vi "IMP Driver.vi"(5 "IMP Driver (\"\")":string, 6 "Drv Refnum":T1, 7 "IMP Command":T2, 8 "error in (no error)":errorcluster, 11 "Variant Input":variant) -> (0 "error out":errorcluster, 3 "Variant Output":variant, 4 "dup Drv Refnum":T1)   [LabVIEW 2011]
uses:
  IMP Command.ctl
  IMP Driver Ref.ctl
panel:
  in  "DEBUG?":bool
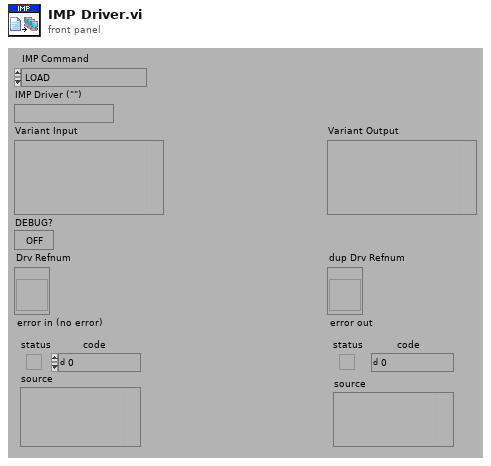
[diagram p1: front panel]
types:
  T1 = typedef "IMP Driver Ref.ctl" = refnum<vi>
  T2 = typedef "IMP Command.ctl" = enum16{"LOAD", "INITIALIZE", "IMPORT", "UNLOAD"}
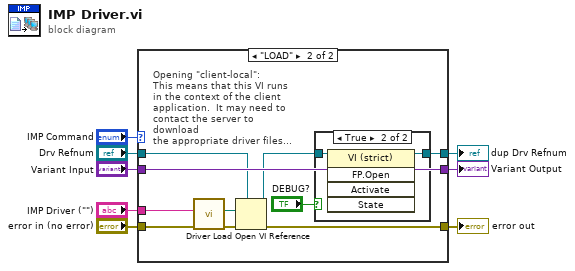
[diagram p0: block diagram]
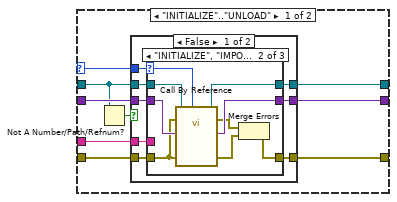
[diagram p2: hidden frame]
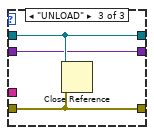
[diagram p4: hidden frame]
diagram:
  n1 = case shown="\"LOAD\"" "IMP Command" {
    selector: "IMP Command" -> [w11 _]
    tunnel: "error in (no error)" -> [w17 w53]
    tunnel: [w16 w52] -> w7
    tunnel: [w15 w51] -> w6
    tunnel: "Drv Refnum" -> [w10 w50]
    tunnel: [w14 w49] -> w4
    tunnel: "IMP Driver (\"\")" -> [w13 w48]
    tunnel: "Variant Input" -> [w12 w52]
    frame "INITIALIZE".."UNLOAD" {
      n2 = Not A Number/Path/Refnum?(number/path/refnum=w10) -> (NaN/Path/Refnum?=w9:bool)
      n3 = case shown="False" w9 {
        tunnel: w17 -> [w25 w41]
        tunnel: [w24 w42] -> w16
        tunnel: [w23 w43] -> w15
        tunnel: w10 -> [w22 w43]
        tunnel: [w21 w41] -> w14
        tunnel: w13 -> [w20 _]
        tunnel: w12 -> [w19 w42]
        tunnel: w11 -> [w18 _]
        frame False {
          n4 = case shown="\"INITIALIZE\", \"IMPORT\"" w18 {
            selector: w18 -> [_ w33 _]
            tunnel: w25 -> [w27 w30 w39]
            tunnel: w19 -> [w28 w34 w38]
            tunnel: [w28 w35 w38] -> w24
            tunnel: [w27 w37 w39] -> w21
            tunnel: w20 -> [_ _ _]
            tunnel: [w26 w36 w40] -> w23
            tunnel: w22 -> [w26 w29 w40]
            frame "LOAD", Default {
              # "This will not ever run."
            }
            frame "INITIALIZE", "IMPORT" {
              n5 = call-by-ref "?"(reference=w29, error in=w30, "IMP Command"=w33, "error in (no error)"=w30, "Variant Input"=w34) -> (reference out=w36:T1, error out=w32:errorcluster, 0:"error out"=w31:errorcluster, "Variant Output"=w35:variant)  [unwired: 7 in]
              n6 = Merge Errors(w32, w31) -> (w37:errorcluster)
            }
            frame "UNLOAD" {
              n7 = Close Reference(reference=w40, error in (no error)=w39) -> ()  [unwired: 1 out]
            }
          }
        }
        frame True {
          # "If the reference is not valid\nno operation is performed."
        }
      }
    }
    frame "LOAD" {
      # "Opening \"client-local\":\nThis means that this VI runs\nin the context of the client\napplication.  It may need to\ncontact the server to download\nthe appropriate driver files..."
      n8 = call "Driver Load.vi"("error in (no error)"=w53, "DriverID DriverType (\"\")"=w48) -> ("error out"=w46:errorcluster, "Driver Component Path"=w45:path)  [unwired: 1 in, 7 out]
      n9 = Open VI Reference(type specifier VI Refnum (for type only)=w50, vi path=w45, error in (no error)=w46) -> (vi reference=w44:T1, error out=w49:errorcluster)  [unwired: 3 out]
      n10 = case shown="True" "DEBUG?" {
        tunnel: w44 -> [w54 w56]
        tunnel: [w54 w55] -> w51
        frame False {
        }
        frame True {
          n11 = invoke class="VI (strict)" method="FP.Open"(reference=w56) -> (reference out=w55:T1)  [unwired: 4 in, 4 out]
        }
      }
    }
  }
  "error out" <- w4
  "Variant Output" <- w7
  "dup Drv Refnum" <- w6
